vi "U32arraytoU8array.vi"(1 "ArrayU32":u32[](array[numeric]) format="%x") -> (0 "ArrayU8":u8[](array[numeric]) format="%x")   [LabVIEW 2015, in "VIPM2.lvlib"]
uses:
  VIPM2.lvlib
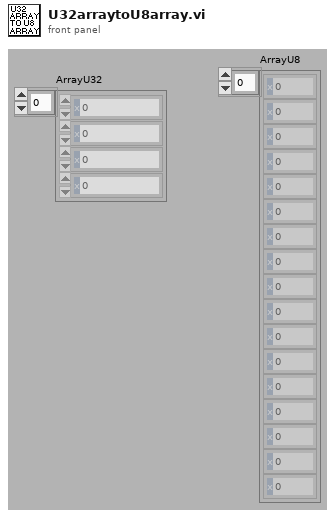
[diagram p1: front panel]
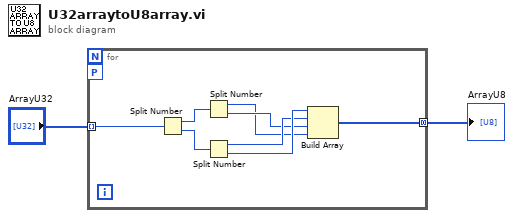
[diagram p0: block diagram]
diagram:
  n1 = for {
    tunnel: "ArrayU32" -> [w10] mode=indexing
    tunnel: [w3] -> w1 mode=concatenating
    workers-P: _ -> [_]
    n2 = Split Number(x=w10) -> (hi(x)=w9:u16, lo(x)=w8:u16)
    n3 = Split Number(x=w9) -> (hi(x)=w4:u8, lo(x)=w5:u8)
    n4 = Split Number(x=w8) -> (hi(x)=w6:u8, lo(x)=w7:u8)
    n5 = Build Array "Build Array"(w7, w6, w5, w4) -> (w3:u8[])
  }
  "ArrayU8" <- w1
